vi "Drag and Drop - Passing Custom Drag Data.vi"() -> ()   [LabVIEW 2023]
doc: "This VI illustrates the use of a built-in Drag and Drop source with custom Drag and Drop data and a custom target. The specific events illustrated by this example are:\n\nDrag Starting? - Triggered when a drag begins. This is a source-side event. Drag Data is passed as an array of 2-element clusters containing a \"data name\" and variant \"drag data.\"\n\nDrag Enter - Triggered when a Drag and Drop enters any control or indicator. This is a target-side event. The Available Data Names are searched for a name that matches the expected data name. If a match is found the Drag enter is accepted and the cursor is changed to indicate that a valid drop target has been found.\n\nDrop - Triggered when a Drag and Drop ends within a control or indicator. This is a target-side event. A Drag and Drop \"data name\" and \"data type\" prototype are given to extract the original data from the array and convert from variant to the intended data type. The Get Drag Drop Data function is used for this process."
panel:
  in  "Signals":i32(listbox)
  in  "Stop":bool
  out "Waveform Graph":dbl[](graph)
  # "Overview: Demonstrates the use of the Event Structure to pass custom data when a Drag and Drop action is initiated on a control.\nInstructions:\n1. Run the VI.\n2. Drag a signal value from the Signals listbox to the Waveform Graph.\n3. Click Stop to stop the VI."
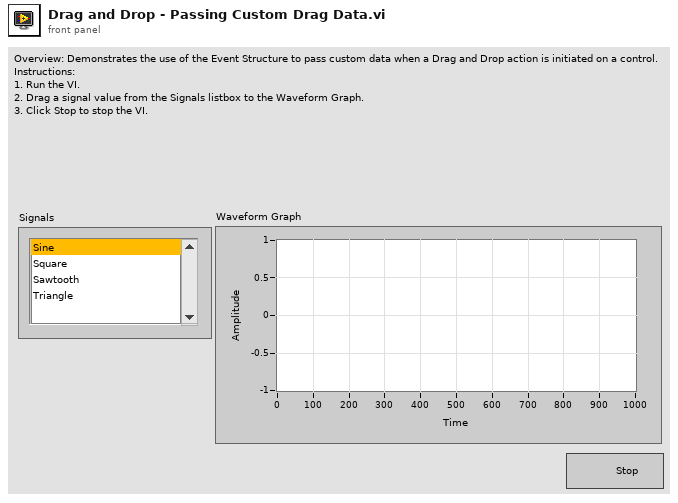
[diagram p1: front panel]
types:
  T1 = cluster{"data name":string, "drag data":variant}[]
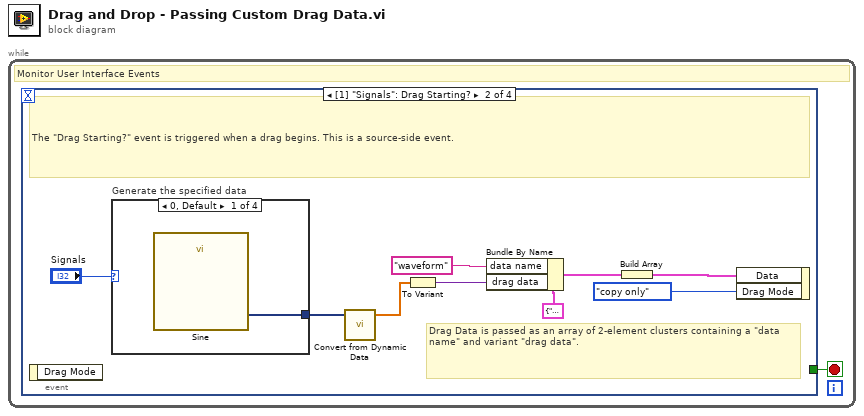
[diagram p0: block diagram]
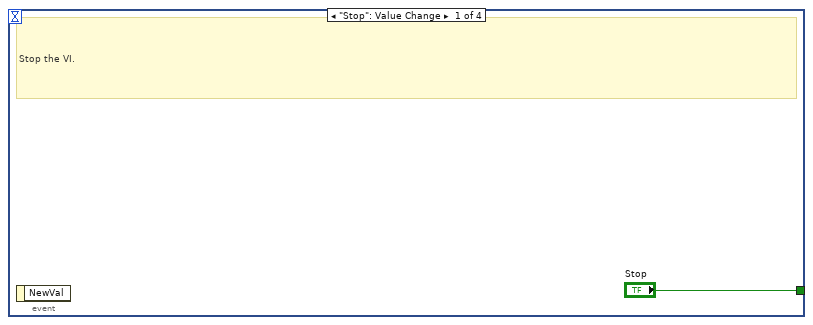
[diagram p2: hidden frame]
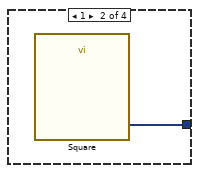
[diagram p3: hidden frame]
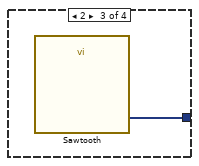
[diagram p4: hidden frame]
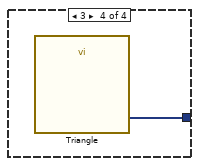
[diagram p5: hidden frame]
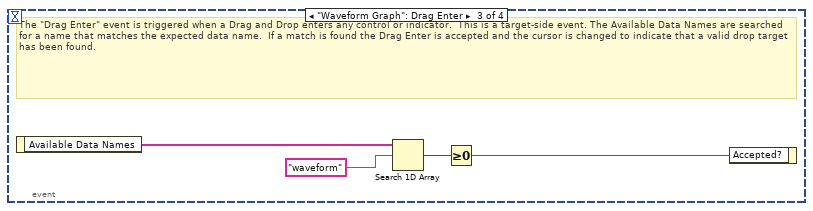
[diagram p6: hidden frame]
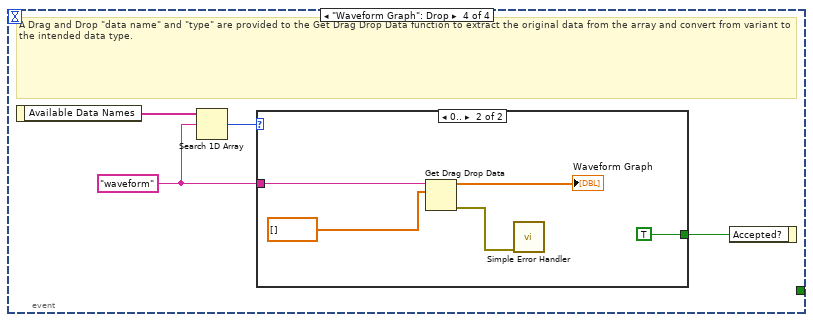
[diagram p7: hidden frame]
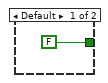
[diagram p8: hidden frame]
diagram:
  n1 = while {
    stop <- w1 stop-if-true
    # "Monitor User Interface Events"
    n2 = event shown="[1] \"Signals\": Drag Starting?" {
      selector: _ -> [_ _ _ _]
      dyn-events: _ -> [_ _ _ _]
      timeout: _ -> [_ _ _ _]
      tunnel: ["Stop" _ _ _] -> w1
      event "Stop": Value Change {
        # "Stop the VI."
        n3 = event-data() -> ()  [unwired: 1 in, 1 out]
      }
      event "Signals": Drag Starting? {
        # "Drag Data is passed as an array of 2-element clusters containing a \"data name\" and variant \"drag data\"."
        # "The \"Drag Starting?\" event is triggered when a drag begins. This is a source-side event."
        n4 = event-data() -> ()  [unwired: 1 in, 1 out]
        n5 = case "Generate the specified data" shown="0, Default" "Signals" {
          tunnel: [w12 w13 w14 w15] -> w4
          frame 0, Default {
            n6 = call "Sine"() -> ("Sine"=w12:dynamicdata)  [unwired: 14 in, 1 out]
          }
          frame 1 {
            n7 = call "Square"() -> ("Square"=w13:dynamicdata)  [unwired: 14 in, 1 out]
          }
          frame 2 {
            n8 = call "Sawtooth"() -> ("Sawtooth"=w14:dynamicdata)  [unwired: 14 in, 1 out]
          }
          frame 3 {
            n9 = call "Triangle"() -> ("Triangle"=w15:dynamicdata)  [unwired: 14 in, 1 out]
          }
        }
        n10 = call "Convert from Dynamic Data"("Dynamic Data Type"=w4) -> ("Array"=w3:dbl[])  [unwired: 3 in]
        n11 = To Variant(anything=w3) -> (Variant=w10:variant)
        n12 = Bundle By Name(cluster=cluster{"data name":string, "drag data":variant} {"data name"="", "drag data"=variant}, "data name"="waveform", "drag data"=w10) -> (w8:cluster{"data name":string, "drag data":variant})
        n13 = Build Array(w8) -> (w7:T1)
        n14 = event-data("Data"=w7, "Drag Mode"=enum32{"copy or move", "copy only", "move only"}."copy only") -> ()  [unwired: 1 in, 1 out]
      }
      event "Waveform Graph": Drag Enter {
        # "The \"Drag Enter\" event is triggered when a Drag and Drop enters any control or indicator.  This is a target-side event. The Available Data Names are searched for a name that matches the expected data name.  If a match is found the Drag Enter is accepted and the cursor is changed to indicate that a valid drop target has been found."
        n15 = event-data() -> ("Available Data Names"=w19:string[])  [unwired: 1 in]
        n16 = Search 1D Array(1D array=w19, element="waveform") -> (index of element=w16:i32)  [unwired: 1 in]
        n17 = Greater Or Equal To 0?(x=w16) -> (x >= 0?=w17:bool)
        n18 = event-data("Accepted?"=w17) -> ()  [unwired: 1 in, 1 out]
      }
      event "Waveform Graph": Drop {
        w20 = "waveform" ("element")
        # "A Drag and Drop \"data name\" and \"type\" are provided to the Get Drag Drop Data function to extract the original data from the array and convert from variant to the intended data type."
        n19 = event-data() -> ("Available Data Names"=w23:string[])  [unwired: 1 in]
        n20 = Search 1D Array(1D array=w23, element=w20) -> (index of element=w21:i32)  [unwired: 1 in]
        n21 = case shown="0.." w21 {
          tunnel: [FALSE TRUE] -> w22
          tunnel: w20 -> [_ w25]
          frame Default {
          }
          frame 0.. {
            n22 = Get Drag Drop Data(8:dbl[] [], 9:w25) -> (0:w26:errorcluster, 3:→"Waveform Graph":dbl[])  [unwired: 1 in]
            n23 = call <vilib>:"Simple Error Handler.vi"("error in (no error)"=w26) -> ()  [unwired: 4 in, 5 out]
          }
        }
        n24 = event-data("Accepted?"=w22) -> ()  [unwired: 1 in, 1 out]
      }
    }
  }
